vi "Add.vi"(9 "Value":string, 10 "Key":string, 11 "Supported Objects in":refnum<class "Supported Objects.lvclass">) -> (3 "Supported Objects out":refnum<class "Supported Objects.lvclass">)   [LabVIEW 2024, in "EDS.lvlib" / "Supported Objects.lvclass"]
uses:
  Supported Objects.lvclass
  Supported Objects.lvclass/Supported Objects.ctl
  EDS.lvlib
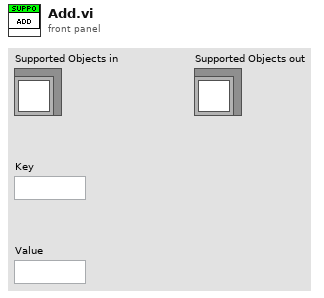
[diagram p1: front panel]
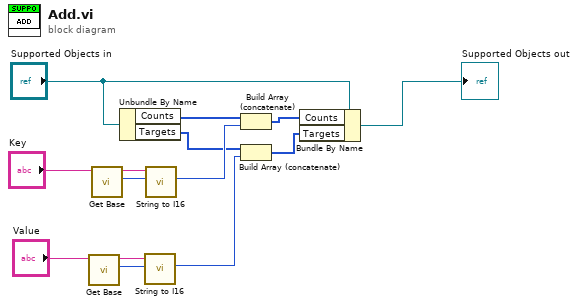
[diagram p0: block diagram]
diagram:
  n1 = call "Get Base.vi"("Default Value"="Value") -> ("Number Base"=w7:u8, "Default Value (dup)"=w8:string)  [unwired: 9 in]
  n2 = call "Get Base.vi"("Default Value"="Key") -> ("Number Base"=w9:u8, "Default Value (dup)"=w10:string)  [unwired: 9 in]
  n3 = Unbundle By Name("Supported Objects in") -> ("Counts"=w6:i16[], "Targets"=w3:i16[])
  n4 = call "String to I16.vi"("Base Number"=w7, "String"=w8) -> ("I16"=w2:i16)  [unwired: 9 in]
  n5 = call "String to I16.vi"("Base Number"=w9, "String"=w10) -> ("I16"=w5:i16)  [unwired: 9 in]
  n6 = Build Array (concatenate)(w6, w5) -> (w4:i16[])
  n7 = Build Array (concatenate)(w3, w2) -> (w1:i16[])
  n8 = Bundle By Name(cluster="Supported Objects in", "Counts"=w4, "Targets"=w1) -> (→"Supported Objects out":refnum<class "Supported Objects.lvclass">)
